vi "Configure Ramp Symmetry.vi"(8 "error in (no error)":errorcluster, 9 "Ramp Symmetry (50.00 %)":dbl=50.0 min=0.0 max=100.0 step=1.0 format="%.2f", 10 "Channel (0: Channel 1)":T1 items=["Channel 1", "Channel 2"], 11 "VISA resource name":refnum<visa-resource-name>) -> (0 "error out":errorcluster, 3 "VISA resource name out":refnum<visa-resource-name>)   [LabVIEW 2023, in "Tektronix AFG 3000 Series.lvlib"]
doc: "Configures the ramp symmetry for Ramp waveforms."
uses:
  Tektronix AFG 3000 Series.lvlib
  controls.llb/Channel.ctl
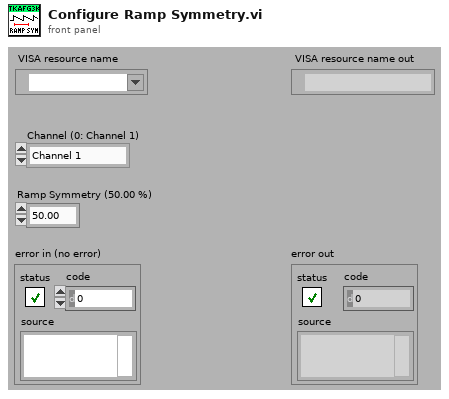
[diagram p1: front panel]
types:
  T1 = typedef "Channel.ctl" = u16
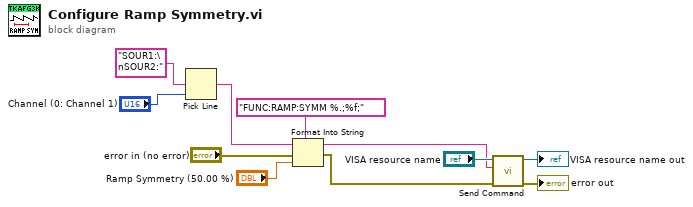
[diagram p0: block diagram]
diagram:
  n1 = Pick Line(multi-line string="SOUR1:\nSOUR2:" ("string (\"\")"), line index="Channel (0: Channel 1)") -> (output string=w7:string)  [unwired: 1 out]
  n2 = Format Into String(format string="FUNC:RAMP:SYMM %.;%f;", initial string=w7, error in="error in (no error)", "Ramp Symmetry (50.00 %)") -> (resulting string=w1:string, error out=w2:errorcluster)
  n3 = call "Send Command.vi"("error in (no error)"=w2, "write buffer"=w1, "VISA resource name"="VISA resource name") -> ("error out"=→"error out":errorcluster, "VISA resource name out"=→"VISA resource name out":refnum<visa-resource-name>)  [unwired: 7 out]
